vi "test.vi"() -> ()   [LabVIEW 2020]
uses:
  splash_screen/splash_screen.lvlib
panel:
  out "String":string
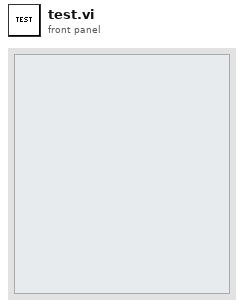
[diagram p1: front panel]
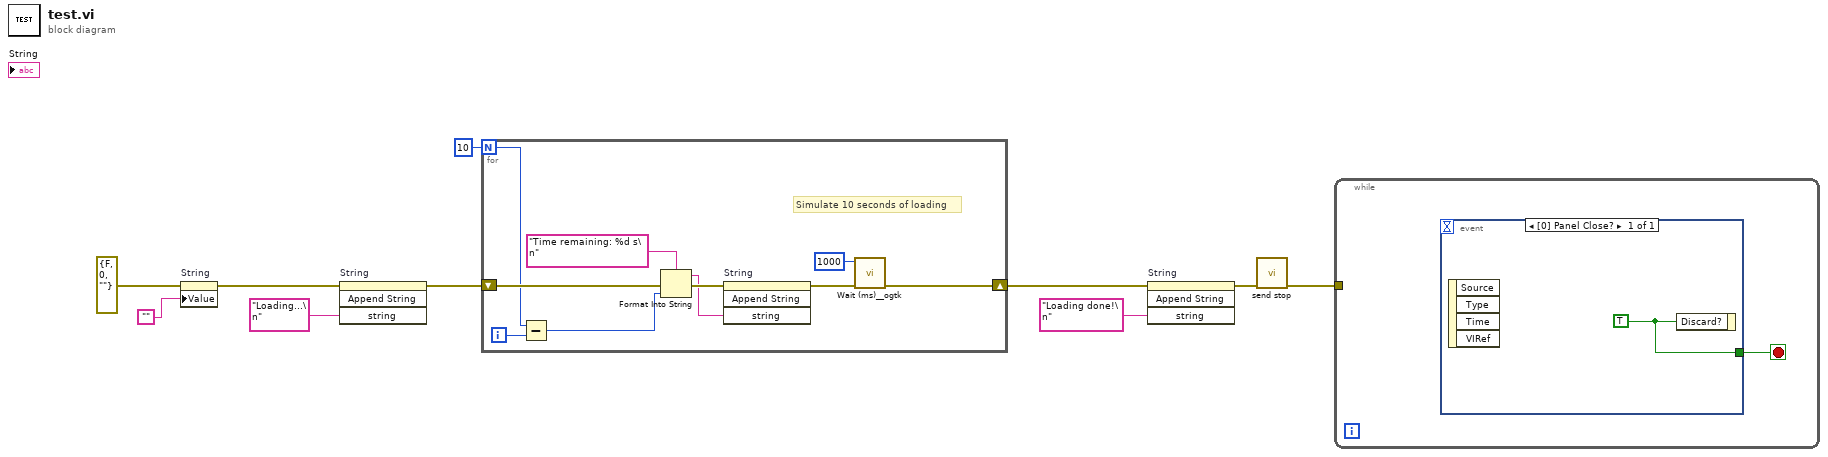
[diagram p0: block diagram]
diagram:
  n1 = property on="String" class="Str"(error in=errorcluster {"status"=FALSE, "code"=0, "source"=""} ("error in (no error)"), "Value"="") -> (error out=w2:errorcluster)  [unwired: 1 in, 1 out]
  n2 = invoke on="String" class="Str" method="Append String"(error in=w2, "string"="Loading...\n" ("String")) -> (error out=w7:errorcluster)  [unwired: 2 in, 3 out]
  n3 = for {
    N: 10 -> [w16]
    shift-right: [w18] -> w6
    shift-left: w7 -> [w19]
    i -> [w17]
    # "Simulate 10 seconds of loading"
    n4 = Subtract(x=w16, y=w17) -> (x-y=w14:i32)
    n5 = Format Into String(format string="Time remaining: %d s\n", error in=w19, w14) -> (resulting string=w12:string, error out=w13:errorcluster)  [unwired: 1 in]
    n6 = invoke on="String" class="Str" method="Append String"(error in=w13, "string"=w12) -> (error out=w11:errorcluster)  [unwired: 2 in, 3 out]
    n7 = call <userlib>:"Wait (ms)__ogtk.vi"("error in (no error)"=w11, "milliseconds to wait"=u32 1000) -> ("error out"=w18:errorcluster)  [unwired: 8 in, 1 out]
  }
  n8 = invoke on="String" class="Str" method="Append String"(error in=w6, "string"="Loading done!\n" ("String")) -> (error out=w4:errorcluster)  [unwired: 2 in, 3 out]
  n9 = call "send stop.vi"("error in (no error)"=w4) -> ("error out"=w10:errorcluster)  [unwired: 10 in]
  n10 = while {
    tunnel: w10 -> [_]
    stop <- w21 stop-if-true
    n11 = event shown="[0] Panel Close?" {
      selector: _ -> [_]
      dyn-events: _ -> [_]
      timeout: _ -> [_]
      tunnel: [w22] -> w21
      event Panel Close? {
        w22 = TRUE
        n12 = event-data() -> ()  [unwired: 1 in, 4 out]
        n13 = event-data("Discard?"=w22) -> ()  [unwired: 1 in, 1 out]
      }
    }
  }
